vi "GEMM_Top.vi"() -> ()   [LabVIEW 2020]
doc: "This benchmark is designed to demonstrate execution performance improvement when executing FFT and IFFT operations on a GPU."
uses:
  <vilib>/Analysis/baseanly.llb/Mean (DBL).vi
  <vilib>/Analysis/1siggen.llb/Ramp Pattern by Delta.vi
  <vilib>/Utility/file.llb/Read Delimited Spreadsheet (DBL).vi
  <vilib>/Ngene/CuLab - GPU Accelerated Toolkit/Toolkit/CuLab.lvlib
  <vilib>/Analysis/NI_AALBase.lvlib
panel:
  in  "CPU Iteration":i32=3
  out "CuLab Mean Performance Gain":dbl[](array[numeric])=[1.0, 32.70718635151803, 2.5525467614410227] format="%#.2g"
  out "Releative Exec Time vs CuLab (smaller is better)":cluster{i32[], "all rows":dbl[]}[](graph)=[{[64, 128, 256, 512, 1024, 2048, 4096, 8192], "all rows"=[1.0, 1.0, 1.0, 1.0, 1.0, 1.0, 1.0, 1.0]}, {[64, 128, 256, 512, 1024, 2048, 4096, 8192], "all rows"=[0.2133838298871944, 1.4083191819921286, 3.1841059555062183, 8.844266159971816, 21.725846108107117, 43.56006909698582, 73.31376485796767, 109.40773562172632]}, {[64, 128, 256, 512, 1024, 2048, 4096, 8192], "all rows"=[7.09343425544868, 4.483870959156996, 1.9112582757762941, 1.4608305799968355, 1.356595313756594, 1.4699518137900995, 1.3925360760265713, 1.251896817576111]}]
  in  "CuPy CSV":path=path "D:/Ngene/GitHub/culab_examples/Benchmarks/CuPy/results/GeForce_RTX_2080_Ti/GEMM_CuPy.csv"
  out "Execution Time":cluster{i32[], "all rows":dbl[]}[](graph)=[{[64, 128, 256, 512, 1024, 2048, 4096, 8192], "all rows"=[3.960000049119117e-05, 5.890000011277152e-05, 0.00015100000018719584, 0.00042380000013508834, 0.0013828000001012697, 0.005499500000041735, 0.02617389999977604, 0.1437802999998894]}, {[64, 128, 256, 512, 1024, 2048, 4096, 8192], "all rows"=[8.449999768345151e-06, 8.294999997815466e-05, 0.00048079999987749034, 0.0037481999997908133, 0.03004250000049069, 0.2395586000006915, 1.9189071499995407, 15.730677050000395]}, {[64, 128, 256, 512, 1024, 2048, 4096, 8192], "all rows"=[0.0002809, 0.0002641, 0.0002886, 0.0006191, 0.0018759000000000002, 0.008084000000000001, 0.036448100000000004, 0.17999810000000002]}]
  out "GPU Model":string="NVIDIA GeForce RTX 2080 Ti"
  out "CPU Model":string="Intel(R) Core(TM) i7-8700K"
  in  "GPU Iteration":i32=50
  in  "Size Stop(2^n)":i32=13
  in  "Size Start(2^n)":i32=6
  out "Dims H,W":i32[](array[numeric])=[64, 128, 256, 512, 1024, 2048, 4096, 8192] format="%.2p"
  # "GEMM Benchmark"
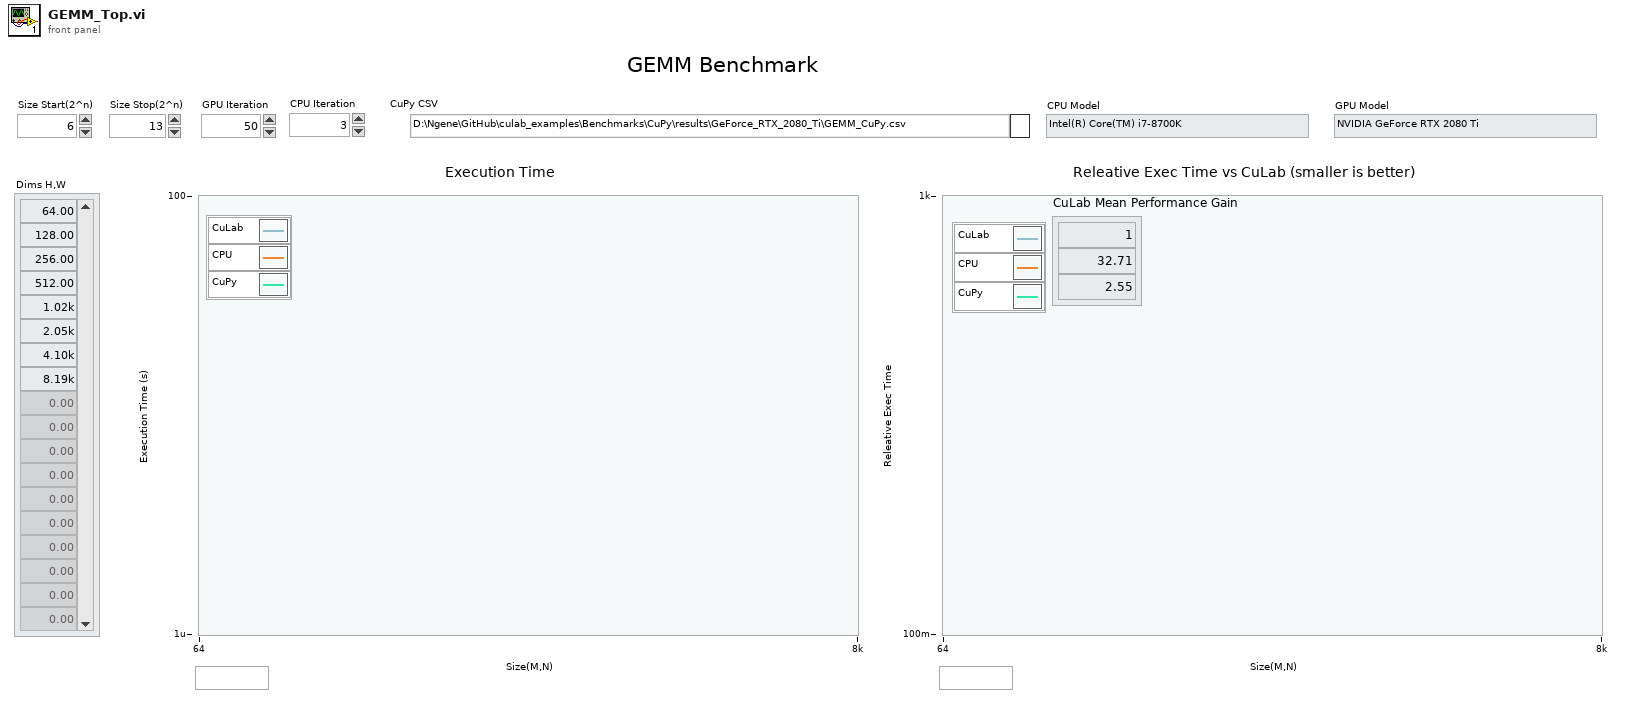
[diagram p1: front panel]
types:
  T1 = typedef "CuLab.lvlib/Properties.ctl" = cluster{"Device ID":i32, "Name":string}
  T2 = typedef "imagedata.ctl" = cluster{"image type":i32, "image depth":i32, "image":u8[], "mask":u8[], "colors":u32[], "Rectangle":cluster{"left":i16, "top":i16, "right":i16, "bottom":i16}}
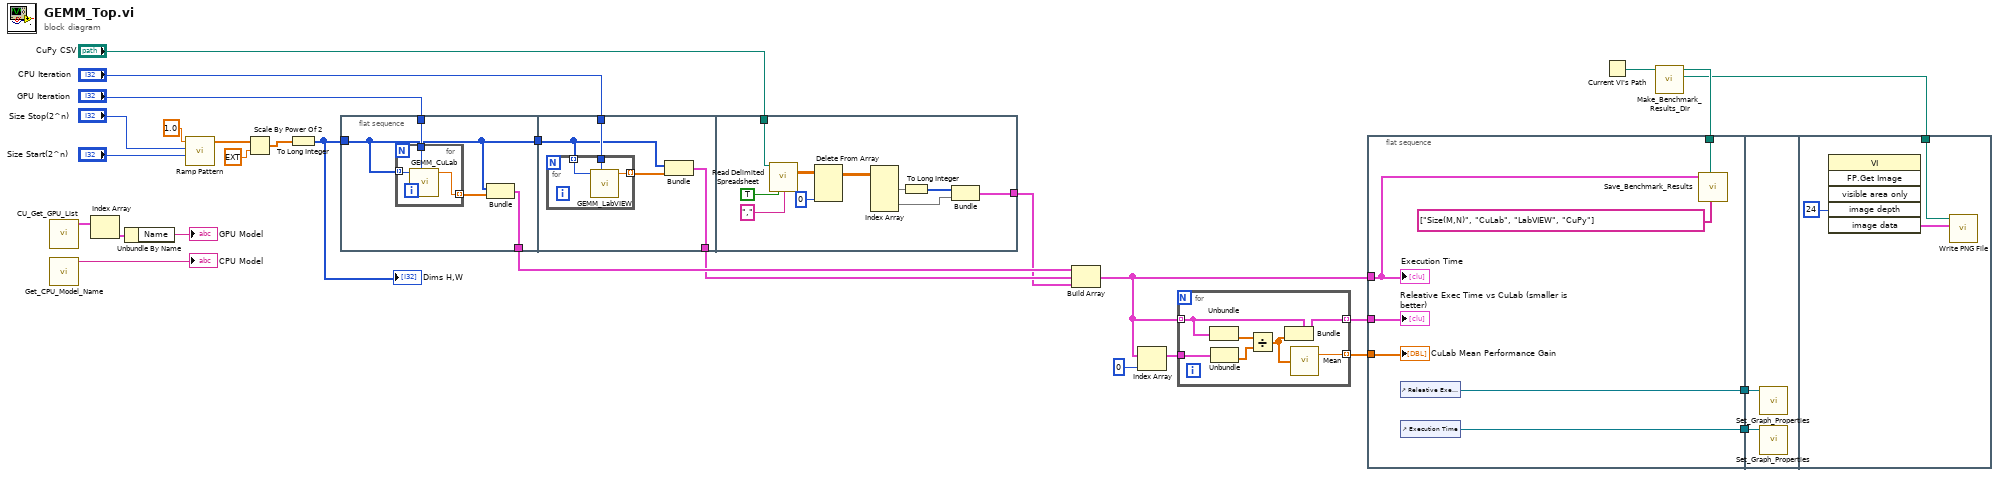
[diagram p0: block diagram]
diagram:
  n1 = call <vilib>:"CU_Get_GPU_List.vi"() -> ("Devices"=w27:T1[])  [unwired: 10 in, 1 out]
  n2 = call "Get_CPU_Model_Name.vi"() -> ("CPU Model"=→"CPU Model":string)  [unwired: 11 in]
  n3 = Index Array(array=w27) -> (element=w26:T1)  [unwired: 1 in]
  n4 = Unbundle By Name(w26) -> ("Name"=→"GPU Model":string)
  n5 = call-poly <vilib>:"Ramp Pattern.vi"("start"="Size Start(2^n)", "end"="Size Stop(2^n)", "delta"=1.0) -> ("Ramp Pattern"=w10:dbl[])  [unwired: 6 in, 2 out]
  n6 = Scale By Power Of 2(n=w10, x=ext 1.0) -> (x*2^n=w12:ext[])
  n7 = To Long Integer(number=w12) -> (32bit integer=w9:i32[])
  "Dims H,W" <- w9
  n8 = flat-sequence {
    tunnel: [w29] -> w24
    tunnel: [w30] -> w25
    tunnel: w9 -> [w30]
    tunnel: "GPU Iteration" -> [w32]
    tunnel: w25 -> [w37]
    tunnel: "CPU Iteration" -> [w39]
    tunnel: [w36] -> w23
    tunnel: "CuPy CSV" -> [w52]
    tunnel: [w44] -> w19
    frame #0 {
      n9 = for {
        tunnel: w32 -> [w33]
        tunnel: w30 -> [w34] mode=indexing
        tunnel: [w35] -> w31 mode=indexing
        n10 = call "GEMM_CuLab.vi"("Iteration"=w33, "Size"=w34) -> ("Result(s)"=w35:dbl)  [unwired: 9 in]
      }
      n11 = Bundle(w30, w31) -> (w29:cluster{i32[], dbl[]})  [unwired: 1 in]
    }
    frame #1 {
      n12 = for {
        tunnel: w37 -> [w42] mode=indexing
        tunnel: w39 -> [w40]
        tunnel: [w41] -> w38 mode=indexing
        n13 = call "GEMM_LabVIEW.vi"("Iteration"=w40, "Size"=w42) -> ("Result(s)"=w41:dbl)  [unwired: 9 in]
      }
      n14 = Bundle(w37, w38) -> (w36:cluster{i32[], dbl[]})  [unwired: 1 in]
    }
    frame #2 {
      n15 = call-poly <vilib>:"Read Delimited Spreadsheet.vi"("file path (dialog if empty)"=w52, "transpose? (F)"=TRUE, "delimiter (\\t)"="," ("delimiter (\\t)")) -> ("all rows"=w50:dbl[][])  [unwired: 7 in, 5 out]
      n16 = Delete From Array(array=w50, index (col)=0 ("disabled index (col)")) -> (array with subset deleted=w48:dbl[][])  [unwired: 2 in, 1 out]
      n17 = Index Array(array=w48) -> (element #1=w47:dbl[], element #2=w45:dbl[])  [unwired: 4 in]
      n18 = To Long Integer(number=w47) -> (32bit integer=w46:i32[])
      n19 = Bundle(w46, "all rows"=w45) -> (w44:cluster{i32[], "all rows":dbl[]})  [unwired: 1 in]
    }
  }
  n20 = Build Array(w24, w23, w19) -> (w16:cluster{i32[], "all rows":dbl[]}[])
  n21 = Index Array(array=w16, index=0) -> (element=w22:cluster{i32[], "all rows":dbl[]})
  n22 = for {
    tunnel: w16 -> [w59] mode=indexing
    tunnel: w22 -> [w57]
    tunnel: [w58] -> w18 mode=indexing
    tunnel: [w53] -> w17 mode=indexing
    n23 = Unbundle(w59) -> ("all rows"=w56:dbl[])  [unwired: 1 out]
    n24 = Unbundle(w57) -> ("all rows"=w55:dbl[])  [unwired: 1 out]
    n25 = Divide(x=w56, y=w55) -> (x/y=w54:dbl[])
    n26 = Bundle(cluster=w59, "all rows"=w54) -> (w58:cluster{i32[], "all rows":dbl[]})  [unwired: 1 in]
    n27 = call-poly <vilib>:"Mean.vi"("X"=w54) -> ("mean"=w53:dbl)  [unwired: 1 out]
  }
  n28 = flat-sequence {
    tunnel: w18 -> [w66]
    tunnel: w17 -> [w65]
    tunnel: w16 -> [w62]
    tunnel: w4 -> [w63]
    tunnel: [w61] -> w2
    tunnel: [w60] -> w1
    tunnel: w2 -> [w68]
    tunnel: w1 -> [w67]
    tunnel: w3 -> [w69]
    frame #0 {
      n29 = control-ref of="Releative Exec Time vs CuLab (smaller is better)"() -> (w61:refnum<vi>)
      n30 = control-ref of="Execution Time"() -> (w60:refnum<vi>)
      n31 = call "Save_Benchmark_Results.vi"("Header"=string[] ["Size(M,N)", "CuLab", "LabVIEW", "CuPy"], "file path (dialog if empty)"=w63, "Execution Time"=w62) -> ()  [unwired: 9 in]
      "Execution Time" <- w62
      "CuLab Mean Performance Gain" <- w65
      "Releative Exec Time vs CuLab (smaller is better)" <- w66
    }
    frame #1 {
      n32 = call "Set_Graph_Properties.vi"("Graph"=w68) -> ()  [unwired: 11 in]
      n33 = call "Set_Graph_Properties.vi"("Graph"=w67) -> ()  [unwired: 11 in]
    }
    frame #2 {
      n34 = invoke class="VI" method="FP.Get Image"("image depth"=24 ("Image Depth")) -> ("image data"=w71:T2)  [unwired: 5 in, 5 out]
      n35 = call <vilib>:"Write PNG File.vi"("image data"=w71, "path to PNG file"=w69) -> ()  [unwired: 8 in, 2 out]
    }
  }
  n36 = Current VI's Path() -> (path=w5:path)
  n37 = call "Make_Benchmark_Results_Dir.vi"("Caller Path"=w5) -> ("Caller FP Image Path"=w3:path, "CSV_File"=w4:path)  [unwired: 9 in]
